vi "WLAN_FrameContent.vi"(11 "Input cluster":cluster{"t0":dbl, "dt":dbl, "Y":cdb[]}) -> (0 "DATA":cdb[](array[numeric]), 1 "SIG":cdb[](array[numeric]), 2 "LTF":cdb[](array[numeric]), 3 "STF":cdb[](array[numeric]))   [LabVIEW 2018]
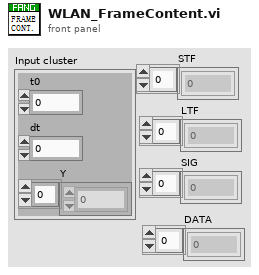
[diagram p1: front panel]
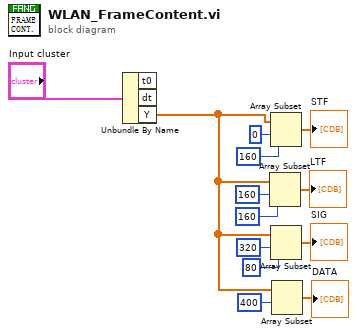
[diagram p0: block diagram]
diagram:
  n1 = Unbundle By Name("Input cluster") -> ("Y"=w13:cdb[])  [unwired: 2 out]
  n2 = Array Subset(array=w13, index=160, length=160) -> (→"LTF":cdb[])
  n3 = Array Subset(array=w13, index=0, length=160) -> (→"STF":cdb[])
  n4 = Array Subset(array=w13, index=320, length=80) -> (→"SIG":cdb[])
  n5 = Array Subset(array=w13, index=400) -> (→"DATA":cdb[])  [unwired: 1 in]
